vi "TCP communication_target.vi"(7 "TCP command":T1(ring), 8 "error in":errorcluster, 9 "remote port":u16=6340, 10 "timeout ms":i32=25000, 11 "data in":string) -> (0 "error out":errorcluster, 3 "Data out":string[](array[string]))   [LabVIEW 2015]
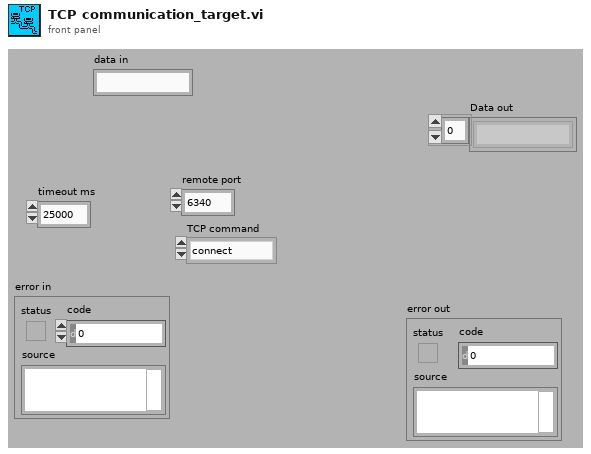
[diagram p1: front panel]
types:
  T1 = enum16{"connect", "receive data", "send data", "data transfer", "close"}
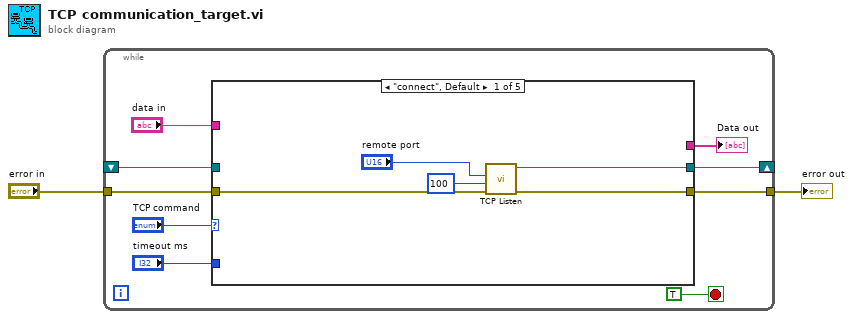
[diagram p0: block diagram]
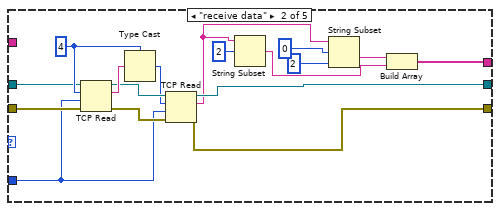
[diagram p2: hidden frame]
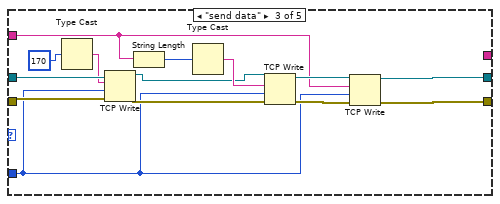
[diagram p3: hidden frame]
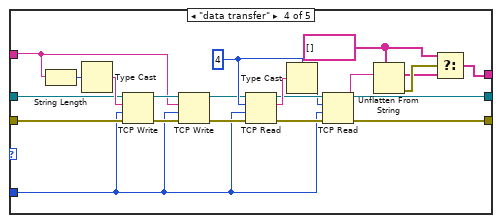
[diagram p4: hidden frame]
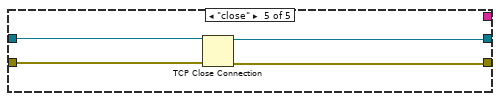
[diagram p5: hidden frame]
diagram:
  n1 = while {
    shift-right: [w11] -> _
    shift-left: _ -> [w9]
    tunnel: "error in" -> [w8]
    tunnel: [w7] -> w1
    stop <- TRUE stop-if-true
    n2 = case shown="\"connect\", Default" "TCP command" {
      tunnel: [w14 w27 w42 w55 w70] -> w11
      tunnel: w9 -> [_ w28 w40 w65 w71]
      tunnel: w8 -> [w12 w26 w37 w64 w73]
      tunnel: [w13 w24 w41 w52 w72] -> w7
      tunnel: [_ w22 _ w48 _] -> w5
      tunnel: "data in" -> [_ _ w43 w63 _]
      tunnel: "timeout ms" -> [_ w25 w34 w53 _]
      frame "connect", Default {
        n3 = call <vilib>:"TCP Listen.vi"("error in (no error)"=w12, "timeout ms (wait forever: -1)"=100 ("timeout ms (60000)"), "port"="remote port") -> ("error out"=w13:errorcluster, "connection ID"=w14:refnum<k5>)  [unwired: 4 in, 3 out]
      }
      frame "receive data" {
        w29 = 4
        n4 = TCP Read(connection ID=w28, bytes to read=w29, error in (no error)=w26, 9:w25) -> (connection ID out=w32:refnum<k5>, data out=w33:string, error out=w31:errorcluster)  [unwired: 1 in]
        n5 = Type Cast(type=w29, x=w33) -> (*(type *) &x=w30:i32)
        n6 = TCP Read(connection ID=w32, bytes to read=w30, error in (no error)=w31, 9:w25) -> (connection ID out=w27:refnum<k5>, data out=w23:string, error out=w24:errorcluster)  [unwired: 1 in]
        n7 = String Subset(string=w23, offset (0)=2) -> (substring=w20:string)  [unwired: 1 in]
        n8 = String Subset(string=w23, offset (0)=0, length (rest)=2 ("length (rest)")) -> (substring=w21:string)
        n9 = Build Array(w21, w20) -> (w22:string[])
      }
      frame "send data" {
        n10 = Type Cast(x=u8 170) -> (*(type *) &x=w35:string)  [unwired: 1 in]
        n11 = TCP Write(connection ID=w40, data in=w35, error in (no error)=w37, 9:w34) -> (connection ID out=w39:refnum<k5>, error out=w38:errorcluster)  [unwired: 1 out]
        n12 = String Length(string=w43) -> (length=w45:i32)
        n13 = Type Cast(x=w45) -> (*(type *) &x=w44:string)  [unwired: 1 in]
        n14 = TCP Write(connection ID=w39, data in=w44, error in (no error)=w38, 9:w34) -> (connection ID out=w47:refnum<k5>, error out=w46:errorcluster)  [unwired: 1 out]
        n15 = TCP Write(connection ID=w47, data in=w43, error in (no error)=w46, 9:w34) -> (connection ID out=w42:refnum<k5>, error out=w41:errorcluster)  [unwired: 1 out]
      }
      frame "data transfer" {
        w49 = string[] [] ("Data In")
        w58 = 4
        n16 = String Length(string=w63) -> (length=w67:i32)
        n17 = Type Cast(x=w67) -> (*(type *) &x=w66:string)  [unwired: 1 in]
        n18 = TCP Write(connection ID=w65, data in=w66, error in (no error)=w64, 9:w53) -> (connection ID out=w69:refnum<k5>, error out=w68:errorcluster)  [unwired: 1 out]
        n19 = TCP Write(connection ID=w69, data in=w63, error in (no error)=w68, 9:w53) -> (connection ID out=w57:refnum<k5>, error out=w56:errorcluster)  [unwired: 1 out]
        n20 = TCP Read(connection ID=w57, bytes to read=w58, error in (no error)=w56, 9:w53) -> (connection ID out=w61:refnum<k5>, data out=w62:string, error out=w60:errorcluster)  [unwired: 1 in]
        n21 = Type Cast(type=w58, x=w62) -> (*(type *) &x=w59:i32)
        n22 = TCP Read(connection ID=w61, bytes to read=w59, error in (no error)=w60, 9:w53) -> (connection ID out=w55:refnum<k5>, data out=w54:string, error out=w52:errorcluster)  [unwired: 1 in]
        n23 = Unflatten From String(type=w49, binary string=w54) -> (value=w50:string[], error out=w51:errorcluster)  [unwired: 3 in, 1 out]
        n24 = Select(t=w49, s=w51, f=w50) -> (s? t:f=w48:string[])
      }
      frame "close" {
        n25 = TCP Close Connection(connection ID=w71, error in (no error)=w73) -> (connection ID out=w70:refnum<k5>, error out=w72:errorcluster)  [unwired: 1 in]
      }
    }
    "Data out" <- w5
  }
  "error out" <- w1
